vi "head.vi"(7 "transmit queue":refnum<queue>, 9 "server information":T1, 10 "application request in":T2, 11 "http responder in":refnum<class "http responder.lvclass">) -> (0 "error out":errorcluster, 3 "http responder out":refnum<class "http responder.lvclass">)   [LabVIEW 2016, in "http responder.lvclass"]
uses:
  http responder.lvclass
  HTTP server/http response.ctl
  HTTP server/http response packet type.ctl
  HTTP headers/http header data.ctl
  HTTP server/http request.ctl
  HTTP server/http method.ctl
  HTTP server/http server info.ctl
  HTTP headers/http add header to set.vi
  HTTP server/Basic HTTP server.lvclass
  HTTP headers/http headers.lvlib
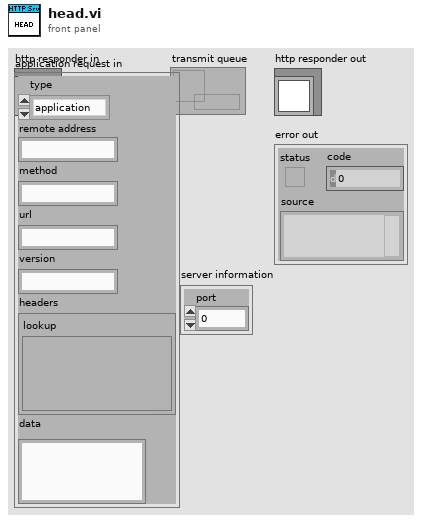
[diagram p1: front panel]
types:
  T1 = typedef "Basic HTTP server.lvclass/http server info.ctl" = cluster{"port":u16}
  T2 = typedef "Basic HTTP server.lvclass/http request.ctl" = cluster{"type":T3, "remote address":string, "method":string, "url":string, "version":string, "headers":T4, "data":string}
  T3 = typedef "Basic HTTP server.lvclass/http method.ctl" = enum16{"application", "error", "upgrade", "expect"}
  T4 = typedef "http headers.lvlib/http header data.ctl" = cluster{"lookup":variant}
  T5 = typedef "Basic HTTP server.lvclass/http response packet type.ctl" = enum16{"full response", "header only", "data only", "last data", "raw output"}
  T6 = typedef "Basic HTTP server.lvclass/http response.ctl" = cluster{"packet type":T5, "reason code":u16, "status string":string, "headers":T4, "cookies":string[], "data":string}
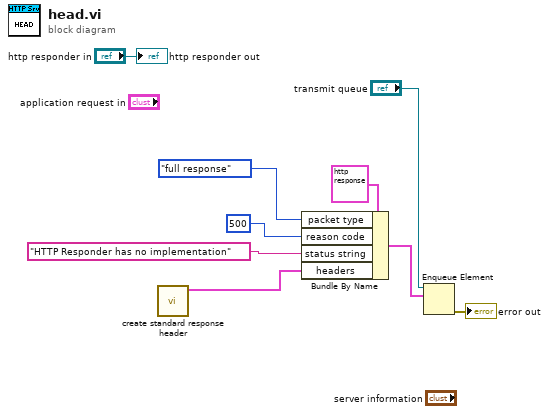
[diagram p0: block diagram]
diagram:
  n1 = call "create standard response header.vi"() -> ("default header"=w1:T4)  [unwired: 11 in]
  n2 = Bundle By Name(cluster=T6 {"packet type"=enum."full response", "reason code"=0, "status string"="", "headers"={"lookup"=variant}, "cookies"=[], "data"=""} ("application request"), "packet type"=http_response_packet_type."full response", "reason code"=u16 500, "status string"="HTTP Responder has no implementation", "headers"=w1) -> (w6:T6)
  n3 = Enqueue Element(queue="transmit queue", element=w6) -> (error out=→"error out":errorcluster)  [unwired: 2 in, 2 out]
  "http responder out" <- "http responder in"
